vi "fonts.vi"() -> ()   [LabVIEW 2015]
uses:
  <vilib>/picture/picture.llb/imagedata.ctl
panel:
  out "filenames":string[](array[string])
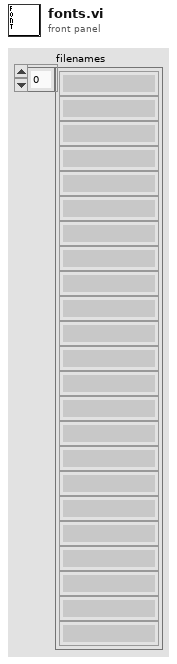
[diagram p1: front panel]
types:
  T1 = typedef "imagedata.ctl" = cluster{"image type":i32, "image depth":i32, "image":u8[], "mask":u8[], "colors":u32[], "Rectangle":cluster{"left":i16, "top":i16, "right":i16, "bottom":i16}}
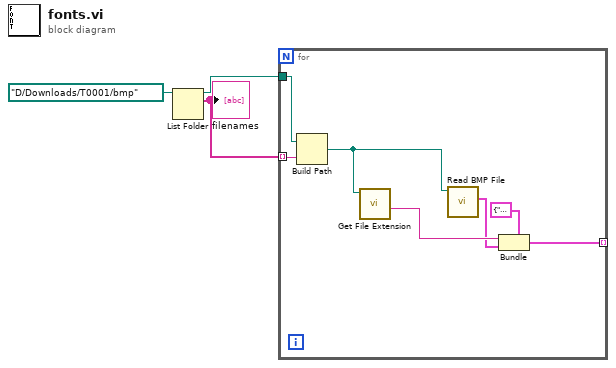
[diagram p0: block diagram]
diagram:
  n1 = List Folder(path=path "D:/Downloads/T0001/bmp") -> (path out=w1:path, filenames=w2:string[])  [unwired: 3 in, 2 out]
  "filenames" <- w2
  n2 = for {
    tunnel: w2 -> [w9] mode=indexing
    tunnel: w1 -> [w10]
    tunnel: [w4] -> _ mode=indexing
    n3 = Build Path(base path=w10, name or relative path=w9) -> (appended path=w8:path)
    n4 = call <vilib>:"Get File Extension.vi"("file"=w8) -> ("filename without extension"=w7:string)  [unwired: 6 in, 4 out]
    n5 = call <vilib>:"Read BMP File.vi"("path to BMP file"=w8) -> ("image data"=w6:T1)  [unwired: 8 in, 2 out]
    n6 = Bundle(cluster=cluster{"font":string, "image data":T1} {"font"="", "image data"={"image type"=0, "image depth"=0, "image"=[], "mask"=[], "colors"=[], "Rectangle"={"left"=0, "top"=0, "right"=0, "bottom"=0}}}, "font"=w7, "image data"=w6) -> (w4:cluster{"font":string, "image data":T1})
  }
